vi "Project2_Navigation_Simulator.vi"() -> ()   [LabVIEW 2016]
panel:
  in  "Sensor 2 Height\n\n                   in":dbl
  in  "Sensor 1 Height\n\n                   in":dbl
  in  "Simulation Timing":dbl
  out "Total Distance":dbl
  out "Sensor 2 Reading":dbl
  out "Sensor 1 Reading":dbl
  out "Angle":dbl
  out "Elapsed Time":dbl
  out "Y Location":dbl
  out "X Location":dbl
  out "Robot Path":cluster{dbl[], dbl[]}[](graph)
  in  "Robot Width":dbl
  in  "Robot Length":dbl
  in  "Run button":bool
  out "2D Picture":picture
  in  "Sensor 2 Mode":u16(ring) items=["Ambient", "Detect", "Reflected"]
  in  "Sensor 1 Mode":u16(ring) items=["Ambient", "Detect", "Reflected"]
  out "Completed?":bool
  out "Average Speed:":dbl
  in  "Sensor 2 Y Location\n\n                    in":dbl
  in  "Sensor 2 X Location\n\n                    in":dbl
  in  "Sensor 1 Y Location\n\n                    in":dbl
  in  "Sensor 1 X Location\n\n                    in":dbl
  in  "Number of \nColor Sensors":u16(ring) items=["1", "2"]
  in  "Select Track":u16(ring) items=["Straight Solid Line", "Straigh Dotted Line", "Straight Broken Line", "Curved Solid Line", "Curved Dotted Line", "Curved Broken Line"]
  # "Setup:"
  # "Status:"
  # "Results:"
  # "s"
  # "in"
  # "in"
  # "ft/s"
  # "in"
  # "in"
  # "degrees"
  # "s"
  # "in"
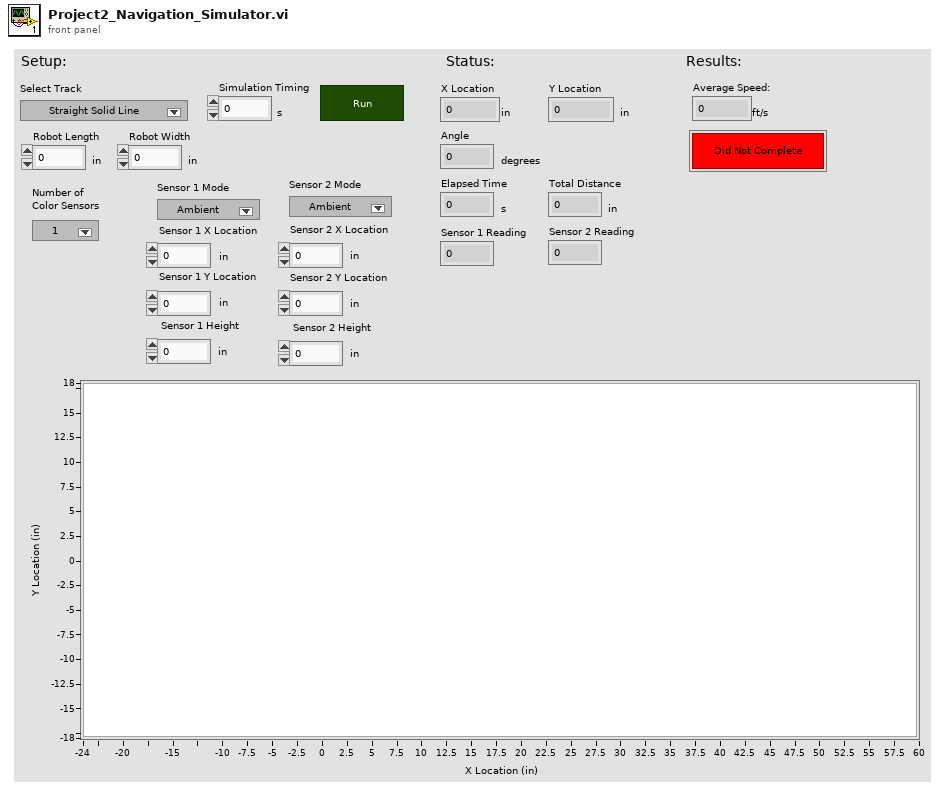
[diagram p1: front panel]
types:
  T1 = typedef "imagedata.ctl" = cluster{"image type":i32, "image depth":i32, "image":u8[], "mask":u8[], "colors":u32[], "Rectangle":cluster{"left":i16, "top":i16, "right":i16, "bottom":i16}}
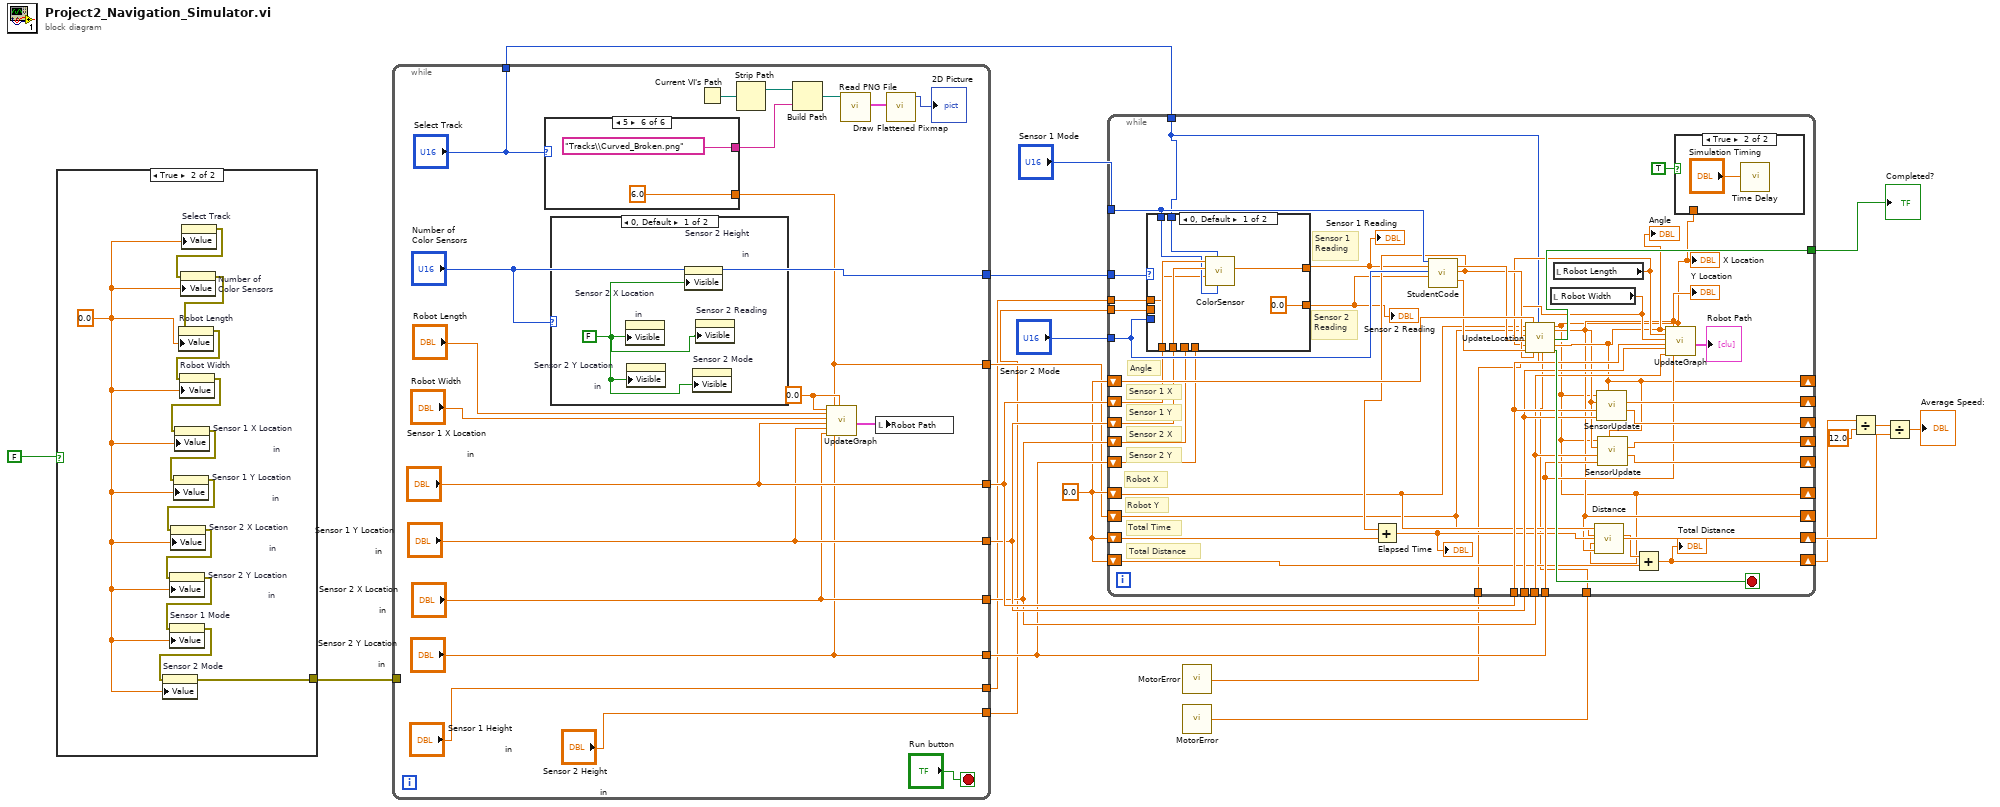
[diagram p0: block diagram]
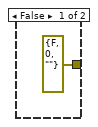
[diagram p2: hidden frame]
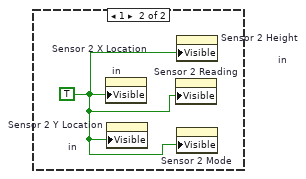
[diagram p3: hidden frame]
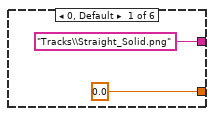
[diagram p4: hidden frame]
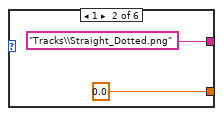
[diagram p5: hidden frame]
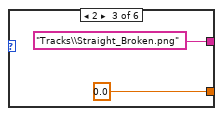
[diagram p6: hidden frame]
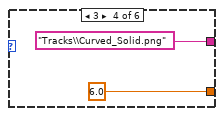
[diagram p7: hidden frame]
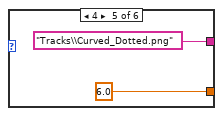
[diagram p8: hidden frame]
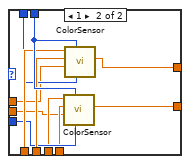
[diagram p10: hidden frame]
diagram:
  w10 = 0.0
  n1 = case shown="True" FALSE {
    tunnel: [errorcluster {"status"=FALSE, "code"=0, "source"=""} ("error out") w24] -> w11
    frame False {
    }
    frame True {
      w34 = 0.0
      n2 = property on="Select Track" class="Ring (strict)"("Value"=w34) -> (error out=w33:errorcluster)  [unwired: 2 in, 1 out]
      n3 = property on="Number of \nColor Sensors" class="Ring (strict)"(error in=w33, "Value"=w34) -> (error out=w32:errorcluster)  [unwired: 1 in, 1 out]
      n4 = property on="Robot Length" class="DigNum (strict)"(error in=w32, "Value"=w34) -> (error out=w31:errorcluster)  [unwired: 1 in, 1 out]
      n5 = property on="Robot Width" class="DigNum (strict)"(error in=w31, "Value"=w34) -> (error out=w30:errorcluster)  [unwired: 1 in, 1 out]
      n6 = property on="Sensor 1 X Location\n\n                    in" class="DigNum (strict)"(error in=w30, "Value"=w34) -> (error out=w29:errorcluster)  [unwired: 1 in, 1 out]
      n7 = property on="Sensor 1 Y Location\n\n                    in" class="DigNum (strict)"(error in=w29, "Value"=w34) -> (error out=w28:errorcluster)  [unwired: 1 in, 1 out]
      n8 = property on="Sensor 2 X Location\n\n                    in" class="DigNum (strict)"(error in=w28, "Value"=w34) -> (error out=w27:errorcluster)  [unwired: 1 in, 1 out]
      n9 = property on="Sensor 2 Y Location\n\n                    in" class="DigNum (strict)"(error in=w27, "Value"=w34) -> (error out=w26:errorcluster)  [unwired: 1 in, 1 out]
      n10 = property on="Sensor 1 Mode" class="Ring (strict)"(error in=w26, "Value"=w34) -> (error out=w25:errorcluster)  [unwired: 1 in, 1 out]
      n11 = property on="Sensor 2 Mode" class="Ring (strict)"(error in=w25, "Value"=w34) -> (error out=w24:errorcluster)  [unwired: 1 in, 1 out]
    }
  }
  n12 = while {
    tunnel: ["Number of \nColor Sensors"] -> w22
    tunnel: ["Select Track"] -> w21
    tunnel: ["Sensor 1 X Location\n\n                    in"] -> w18
    tunnel: ["Sensor 1 Y Location\n\n                    in"] -> w17
    tunnel: ["Sensor 2 X Location\n\n                    in"] -> w16
    tunnel: ["Sensor 2 Y Location\n\n                    in"] -> w15
    tunnel: w11 -> [_]
    tunnel: [w37] -> w5
    tunnel: ["Sensor 1 Height\n\n                   in"] -> w2
    tunnel: ["Sensor 2 Height\n\n                   in"] -> w1
    stop <- "Run button" stop-if-true
    w45 = 0.0 ("Angle")
    n13 = case shown="5" "Select Track" {
      tunnel: ["Tracks\\Straight_Solid.png" "Tracks\\Straight_Dotted.png" "Tracks\\Straight_Broken.png" "Tracks\\Curved_Solid.png" "Tracks\\Curved_Dotted.png" "Tracks\\Curved_Broken.png"] -> w51
      tunnel: [0.0 ("Angle") 0.0 ("Angle") 0.0 ("Angle") 6.0 ("Angle") 6.0 ("Angle") 6.0 ("Angle")] -> w37
      frame 0, Default {
      }
      frame 1 {
      }
      frame 2 {
      }
      frame 3 {
      }
      frame 4 {
      }
      frame 5 {
      }
    }
    n14 = case shown="0, Default" "Number of \nColor Sensors" {
      frame 0, Default {
        w55 = FALSE ("Visible")
        n15 = property on="Sensor 2 X Location\n\n                    in" class="DigNum (strict)"("Visible"=w55) -> ()  [unwired: 2 in, 2 out]
        n16 = property on="Sensor 2 Y Location\n\n                    in" class="DigNum (strict)"("Visible"=w55) -> ()  [unwired: 2 in, 2 out]
        n17 = property on="Sensor 2 Height\n\n                   in" class="DigNum (strict)"("Visible"=w55) -> ()  [unwired: 2 in, 2 out]
        n18 = property on="Sensor 2 Mode" class="Ring (strict)"("Visible"=w55) -> ()  [unwired: 2 in, 2 out]
        n19 = property on="Sensor 2 Reading" class="DigNum (strict)"("Visible"=w55) -> ()  [unwired: 2 in, 2 out]
      }
      frame 1 {
        w56 = TRUE ("Visible")
        n20 = property on="Sensor 2 X Location\n\n                    in" class="DigNum (strict)"("Visible"=w56) -> ()  [unwired: 2 in, 2 out]
        n21 = property on="Sensor 2 Y Location\n\n                    in" class="DigNum (strict)"("Visible"=w56) -> ()  [unwired: 2 in, 2 out]
        n22 = property on="Sensor 2 Reading" class="DigNum (strict)"("Visible"=w56) -> ()  [unwired: 2 in, 2 out]
        n23 = property on="Sensor 2 Height\n\n                   in" class="DigNum (strict)"("Visible"=w56) -> ()  [unwired: 2 in, 2 out]
        n24 = property on="Sensor 2 Mode" class="Ring (strict)"("Visible"=w56) -> ()  [unwired: 2 in, 2 out]
      }
    }
    n25 = Current VI's Path() -> (path=w52:path)
    n26 = Strip Path(path=w52) -> (stripped path=w38:path)  [unwired: 1 out]
    n27 = Build Path(base path=w38, name or relative path=w51) -> (appended path=w50:path)
    n28 = call "UpdateGraph.vi"("Angle"=w45, "Robot Length"="Robot Length", "Robot Width"="Robot Width", "Sensor 1 X"="Sensor 1 X Location\n\n                    in", "Sensor 1 Y"="Sensor 1 Y Location\n\n                    in", "Sensor 2 X"="Sensor 2 X Location\n\n                    in", "Robot Y"=w37, "Sensor 2 Y"="Sensor 2 Y Location\n\n                    in", "Robot X"=w45) -> ("appended array"=w53:cluster{dbl[], dbl[]}[])  [unwired: 10 in]
    n29 = call <vilib>:"Read PNG File.vi"("path to PNG file"=w50) -> ("image data"=w49:T1)  [unwired: 8 in, 2 out]
    n30 = local write "Robot Path"(w53) -> ()
    n31 = call <vilib>:"Draw Flattened Pixmap.vi"("image data"=w49) -> ("new picture"=→"2D Picture":picture)  [unwired: 8 in]
  }
  n32 = call "MotorError.vi"() -> ("Motor Error Value"=w4:dbl)
  n33 = call "MotorError.vi"() -> ("Motor Error Value"=w3:dbl)
  n34 = while {
    shift-right: [w69] -> _
    shift-left: w10 -> [w81]
    shift-right: [w75] -> _
    shift-left: w5 -> [w80]
    tunnel: w22 -> [w109]
    tunnel: w21 -> [w85]
    shift-right: [w106] -> _
    shift-left: w18 -> [w79]
    shift-right: [w105] -> _
    shift-left: w17 -> [w78]
    shift-right: [w104] -> _
    shift-left: w16 -> [w77]
    shift-right: [w103] -> _
    shift-left: w15 -> [w76]
    shift-right: [w86] -> _
    shift-left: w10 -> [w108]
    tunnel: "Sensor 1 Mode" -> [w98]
    tunnel: "Sensor 2 Mode" -> [w97]
    tunnel: w18 -> [w102]
    tunnel: w17 -> [w101]
    tunnel: w16 -> [w100]
    tunnel: w15 -> [w99]
    tunnel: [w94] -> w14
    shift-right: [w89] -> w12
    shift-left: w10 -> [w93]
    shift-right: [w82] -> w9
    shift-left: w10 -> [w84]
    tunnel: w4 -> [w74]
    tunnel: w3 -> [w73]
    tunnel: w2 -> [w72]
    tunnel: w1 -> [w71]
    stop <- w107 stop-if-true
    # "Total Distance"
    # "Total Time"
    # "Sensor 2\nReading"
    # "Sensor 1\nReading"
    # "Sensor 2 Y"
    # "Sensor 2 X"
    # "Sensor 1 Y"
    # "Sensor 1 X"
    # "Angle"
    # "Robot Y"
    # "Robot X"
    n35 = case shown="0, Default" w109 {
      tunnel: [w118 w129] -> w88
      tunnel: [0.0 ("Color Sensor Reading") w128] -> w87
      tunnel: w85 -> [w116 w127]
      tunnel: w79 -> [w115 w125]
      tunnel: w78 -> [w114 w126]
      tunnel: w98 -> [w113 w124]
      tunnel: w97 -> [_ w123]
      tunnel: w77 -> [_ w122]
      tunnel: w76 -> [_ w121]
      tunnel: w72 -> [w112 w120]
      tunnel: w71 -> [_ w119]
      frame 0, Default {
        n36 = call "ColorSensor.vi"("Sensor Mode"=w113, "Select Track"=w116, "Height"=w112, "Y Location Sensor"=w114, "X Location Sensor"=w115) -> ("Color Sensor Reading"=w118:dbl)  [unwired: 6 in]
      }
      frame 1 {
        n37 = call "ColorSensor.vi"("Sensor Mode"=w123, "Select Track"=w127, "Height"=w119, "Y Location Sensor"=w121, "X Location Sensor"=w122) -> ("Color Sensor Reading"=w128:dbl)  [unwired: 6 in]
        n38 = call "ColorSensor.vi"("Sensor Mode"=w124, "Select Track"=w127, "Height"=w120, "Y Location Sensor"=w126, "X Location Sensor"=w125) -> ("Color Sensor Reading"=w129:dbl)  [unwired: 6 in]
      }
    }
    "Sensor 1 Reading" <- w88
    "Sensor 2 Reading" <- w87
    n39 = call "StudentCode.vi"("Sensor 1 Mode"=w98, "Sensor 1 Value"=w88, "Sensor 2 Mode"=w97, "Sensor 2 Value"=w87) -> ("Motor 1 Value"=w96:dbl, "Motor On Duration"=w92:dbl, "Motor 2 Value"=w95:dbl)  [unwired: 13 in]
    n40 = Add(x=w92, y=w93) -> (x+y=w89:dbl)
    "Elapsed Time" <- w89
    n41 = local read "Robot Width"() -> (w91:dbl)
    n42 = local read "Robot Length"() -> (w90:dbl)
    n43 = call "UpdateLocation.vi"("Robot X Location"=w81, "Robot Y Location"=w80, "Robot Width"=w91, "Motor 1 Value"=w96, "Robot Length"=w90, "Motor 2 Value"=w95, "Angle"=w108, "Motor On Duration"=w92, "Select Track"=w85, "Motor 1 Error"=w74, "Motor 2 Error"=w73) -> ("New Robot X Location"=w69:dbl, "New Robot Y Location"=w75:dbl, "Complete?"=w94:bool, "New Angle"=w86:dbl, "Terminate?"=w107:bool)  [unwired: 4 in]
    "X Location" <- w69
    "Y Location" <- w75
    "Angle" <- w86
    n44 = call "Distance.vi"("New y"=w75, "New X"=w69, "Original y"=w80, "Original X"=w81) -> ("Distance"=w83:dbl)  [unwired: 7 in]
    n45 = call "SensorUpdate.vi"("Angle"=w86, "Sensor Y"=w101, "Sensor X"=w102, "Robot Y"=w75, "Robot X"=w69) -> ("New Sensor Y"=w105:dbl, "New Sensor X"=w106:dbl)  [unwired: 5 in]
    n46 = call "SensorUpdate.vi"("Angle"=w86, "Sensor Y"=w99, "Sensor X"=w100, "Robot Y"=w75, "Robot X"=w69) -> ("New Sensor Y"=w103:dbl, "New Sensor X"=w104:dbl)  [unwired: 5 in]
    n47 = Add(x=w83, y=w84) -> (x+y=w82:dbl)
    "Total Distance" <- w82
    n48 = call "UpdateGraph.vi"("Angle"=w86, "Robot Length"=w90, "Robot Width"=w91, "Sensor 1 X"=w102, "Sensor 1 Y"=w101, "Sensor 2 X"=w100, "Robot Y"=w75, "Sensor 2 Y"=w99, "Robot X"=w69) -> ("appended array"=→"Robot Path":cluster{dbl[], dbl[]}[])  [unwired: 10 in]
    n49 = case shown="True" TRUE {
      tunnel: w69 -> [_ _]
      frame False {
      }
      frame True {
        n50 = call "Time Delay"("Delay Time (s)"="Simulation Timing") -> ()  [unwired: 10 in, 1 out]
      }
    }
  }
  "Completed?" <- w14
  n51 = Divide(x=w9, y=12.0) -> (x/y=w8:dbl)
  n52 = Divide(x=w8, y=w12) -> (x/y=→"Average Speed:":dbl)
